vi "simple predict step.vi"(6 "v scaler":u32, 7 "update velocity estimate?":bool, 10 "state in":T1) -> (2 "state out":T1)   [LabVIEW 2010]
uses:
  kalman simple pv state.ctl
  <vilib>/rvi/FXPMathLib/FxpAdd/XNode/nifxpmath_Add.xnode
  <vilib>/rvi/FXPMathLib/FxpAdd/subVIs/nifxpmath_Add_SimConfig.ctl
  <vilib>/fxp/LVFixedPointQuantizationPolicyTypeDef.ctl
  <vilib>/fxp/LVFixedPointOverflowPolicyTypeDef.ctl
  <vilib>/rvi/FXPMathLib/FxpAdd/simVIs/DllFxpAddTemp_sub.vi
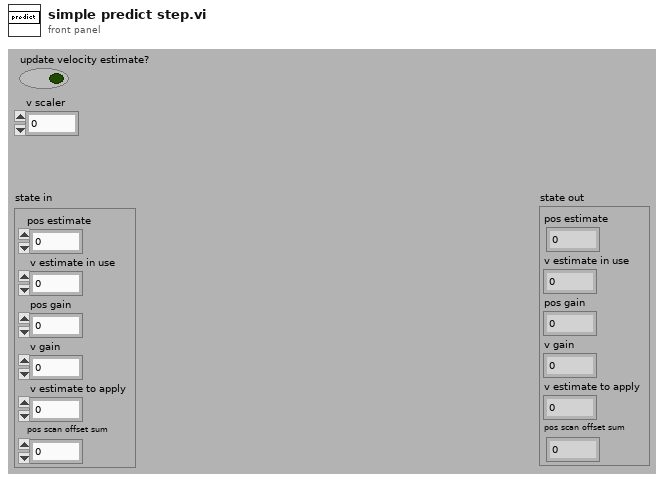
[diagram p1: front panel]
types:
  T1 = typedef "kalman simple pv state.ctl" = cluster{"pos estimate":fxp<+/-,32,16>, "v estimate in use":fxp<+/-,32,-4>, "pos gain":fxp<+,32,0>, "v gain":fxp<+,32,-16>, "v estimate to apply":fxp<+/-,32,-4>, "pos scan offset sum":fxp<+/-,32,35>}
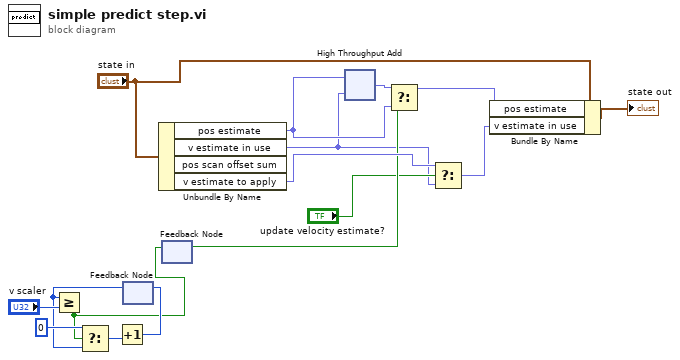
[diagram p0: block diagram]
diagram:
  n1 = feedback #1() -> (w2:u32)  [unwired: 1 in]
  n2 = Greater Or Equal?(x=w2, y="v scaler") -> (x >= y?=w1:bool)
  n3 = Select(t=u32 0, s=w1, f=w2) -> (s? t:f=w5:u32)
  n4 = Increment(x=w5) -> (x+1=w4:u32)
  n5 = feedback-in #1(w4) -> ()
  n6 = Unbundle By Name("state in") -> ("pos estimate"=w9:fxp<+/-,32,16>, "v estimate in use"=w7:fxp<+/-,32,-4>, "v estimate to apply"=w13:fxp<+/-,32,-4>)  [unwired: 1 out]
  n7 = feedback-in #2(w1) -> ()
  n8 = feedback #2() -> (w10:bool)  [unwired: 1 in]
  n9 = xnode "High Throughput Add"("x"=w9, "y"=w7) -> ("x+y"=w15:fxp<+/-,32,16>)
  n10 = Select(t=w15, s=w10, f=w9) -> (s? t:f=w11:fxp<+/-,32,16>)
  n11 = Select(t=w13, s="update velocity estimate?", f=w7) -> (s? t:f=w12:fxp<+/-,32,-4>)
  n12 = Bundle By Name(cluster="state in", "pos estimate"=w11, "v estimate in use"=w12) -> (→"state out":T1)
